vi "Emballage_BDD_SortChaineDunCode2D.vi"(9 "Fin_CHAINE":string, 10 "Debut_CHAINE":string, 11 "Chaine_Lecteur":string) -> (1 "Chaîne OUT":string)   [LabVIEW 2020]
panel:
  out "Sep_Fin":string=";"
  out "Chaîne IN 2":string
  out "Fin":i32
  out "début":i32
  out "Sep_Debut":string=";"
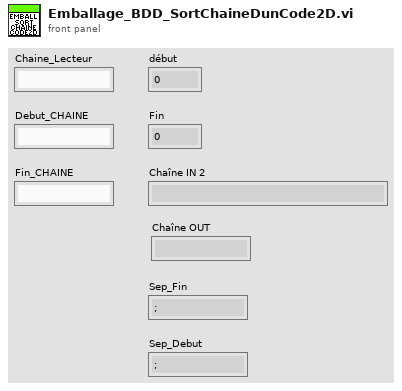
[diagram p1: front panel]
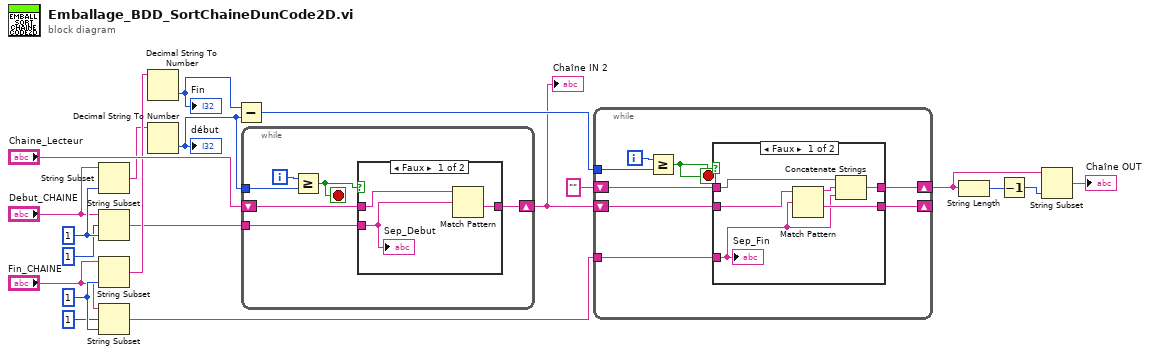
[diagram p0: block diagram]
diagram:
  w19 = 1 ("longueur (reste)")
  w18 = 1 ("longueur (reste)")
  n1 = String Subset(string="Debut_CHAINE", length (rest)=w18) -> (substring=w9:string)  [unwired: 1 in]
  n2 = String Subset(string="Debut_CHAINE", offset (0)=1, length (rest)=w18) -> (substring=w11:string)
  n3 = String Subset(string="Fin_CHAINE", length (rest)=w19) -> (substring=w12:string)  [unwired: 1 in]
  n4 = String Subset(string="Fin_CHAINE", offset (0)=1, length (rest)=w19) -> (substring=w15:string)
  n5 = Decimal String To Number(string=w12) -> (number=w20:i32)  [unwired: 2 in, 1 out]
  "Fin" <- w20
  n6 = Decimal String To Number(string=w9) -> (number=w10:i32)  [unwired: 2 in, 1 out]
  "début" <- w10
  n7 = Subtract(x=w20, y=w10) -> (x-y=w2:i32)
  n8 = while {
    tunnel: w10 -> [w24]
    shift-right: [w25] -> w1
    shift-left: "Chaine_Lecteur" -> [w26]
    tunnel: w11 -> [w21]
    i -> [w23]
    stop <- w22 stop-if-true
    n9 = Greater Or Equal?(x=w23, y=w24) -> (x >= y?=w22:bool)
    n10 = case shown="Faux" w22 {
      tunnel: w26 -> [w29 w30]
      tunnel: [w28 w30] -> w25
      tunnel: w21 -> [w27 _]
      frame False {
        n11 = Match Pattern(string=w29, regular expression=w27) -> (after substring=w28:string)  [unwired: 1 in, 3 out]
        "Sep_Debut" <- w27
      }
      frame True {
      }
    }
  }
  "Chaîne IN 2" <- w1
  n12 = while {
    tunnel: w2 -> [w36]
    shift-right: [w37] -> _
    shift-left: w1 -> [w38]
    shift-right: [w33] -> w4
    shift-left: "" ("Chaîne IN") -> [w32]
    tunnel: w15 -> [w31]
    i -> [w35]
    stop <- w34 stop-if-true
    n13 = Greater Or Equal?(x=w35, y=w36) -> (x >= y?=w34:bool)
    n14 = case shown="Faux" w34 {
      tunnel: w38 -> [w44 w46]
      tunnel: [w43 w46] -> w37
      tunnel: [w42 w45] -> w33
      tunnel: w32 -> [w41 w45]
      tunnel: w31 -> [w39 _]
      frame False {
        n15 = Match Pattern(string=w44, regular expression=w39) -> (before substring=w40:string, after substring=w43:string)  [unwired: 1 in, 2 out]
        n16 = Concatenate Strings(w41, w40, w39) -> (w42:string)
        "Sep_Fin" <- w39
      }
      frame True {
      }
    }
  }
  n17 = String Length(string=w4) -> (length=w5:i32)
  n18 = Decrement(x=w5) -> (x-1=w6:i32)
  n19 = String Subset(string=w4, length (rest)=w6) -> (substring=→"Chaîne OUT":string)  [unwired: 1 in]
